vi "FaulhaberV3-Ascii_V1.vi"() -> (1 "searchnames":string[](array[string]), 2 "ID":u32[](array[numeric]), 3 "Faulhaber Objects":T3(array[cluster]))   [LabVIEW 2011] (continued)
  in  "?":string="<?xml version=\"1.0\" encoding=\"utf-8\"?>\n<ISO15745ProfileContainer xmlns=\"http://www.canopen.org/xml/1.0\" xmlns:xsi=\"http://www.w3.org/2001/XMLSchema-instance\" xsi:schemaLocation=\"http://www.canopen.org/xml/1.0 CANopen.xsd\">\n\t<ISO15745Profile>\n\t\t<ProfileHeader>\n\t\t\t<ProfileIdentification>CAN device profile</ProfileIdentification>\n\t\t\t<ProfileRevision>1</ProfileRevision>\n\t\t\t<ProfileName></ProfileName>\n\t\t\t<ProfileSource></ProfileSource>\n\t\t\t<ProfileClassID>Device</ProfileClassID>\n\t\t\t<ISO15745Reference>\n\t\t\t\t<ISO15745Part>1</ISO15745Part>\n\t\t\t\t<ISO15745Edition>1</ISO15745Edition>\n\t\t\t\t<ProfileTechnology>CANopen</ProfileTechnology>\n\t\t\t</ISO15745Reference>\n\t\t</ProfileHeader>\n\t\t<ProfileBody xsi:type=\"ProfileBody_Device_CANopen\" fileName=\"605.0161.01-O.xdd\" fileCreator=\"Dr. Fritz Faulhaber GmbH &amp; Co KG\" fileCreationDate=\"2024-11-08\" fileCreationTime=\"07:04:39\" fileModificationDate=\"2024-11-08\" fileModificationTime=\"07:04:39\" fileModifiedBy=\"Dr. Fritz Faulhaber GmbH &amp; Co KG\" fileVersion=\"1\" supportedLanguages=\"en\">\n\t\t\t<DeviceIdentity>\n\t\t\t\t<vendorName readOnly=\"true\">Dr. Fritz Faulhaber GmbH &amp; Co KG</vendorName>\n\t\t\t\t<vendorID readOnly=\"true\">327</vendorID>\n\t\t\t\t<vendorText readOnly=\"true\">\n\t\t\t\t\t<label lang=\"en\" />\n\t\t\t\t</vendorText>\n\t\t\t\t<deviceFamily readOnly=\"true\">\n\t\t\t\t\t<label lang=\"en\" />\n\t\t\t\t</deviceFamily>\n\t\t\t\t<productFamily readOnly=\"true\">MC V3.x</productFamily>\n\t\t\t\t<productName readOnly=\"true\">IMC *</productName>\n\t\t\t\t<productID readOnly=\"true\">016101</productID>\n\t\t\t\t<productText readOnly=\"true\">\n\t\t\t\t\t<description lang=\"en\">FileDescription=Faulhaber MC V3.x device description|EdsVersion=4.0|FileRevison=1|RevisionNum=0x00010000|</description>\n\t\t\t\t</productText>\n\t\t\t\t<orderNumber readOnly=\"true\">0</orderNumber>\n\t\t\t\t<version versionType=\"SW\" readOnly=\"true\"></version>\n\t\t\t\t<version versionType=\"FW\" readOnly=\"true\"></version>\n\t\t\t\t<version versionType=\"HW\" readOnly=\"true\"></version>\n\t\t\t\t<specificationRevision readOnly=\"true\"></specificationRevision>\n\t\t\t\t<instanceName readOnly=\"true\"></instanceName>\n\t\t\t</DeviceIdentity>\n\t\t\t<DeviceManager>\n\t\t\t\t<indicatorList>\n\t\t\t\t\t<LEDList>\n\t\t\t\t\t\t<LED LEDcolors=\"monocolor\" LEDtype=\"device\">\n\t\t\t\t\t\t\t<label lang=\"en\" />\n\t\t\t\t\t\t\t<LEDstate uniqueID=\"LED_State_1\" state=\"off\" LEDcolor=\"green\">\n\t\t\t\t\t\t\t\t<label lang=\"en\" />\n\t\t\t\t\t\t\t</LEDstate>\n\t\t\t\t\t\t</LED>\n\t\t\t\t\t</LEDList>\n\t\t\t\t</indicatorList>\n\t\t\t</DeviceManager>\n\t\t\t<DeviceFunction>\n\t\t\t\t<capabilities>\n\t\t\t\t\t<characteristicsList>\n\t\t\t\t\t\t<characteristic>\n\t\t\t\t\t\t\t<characteristicName>\n\t\t\t\t\t\t\t\t<label lang=\"en\" />\n\t\t\t\t\t\t\t</characteristicName>\n\t\t\t\t\t\t\t<characteristicContent>\n\t\t\t\t\t\t\t\t<label lang=\"en\" />\n\t\t\t\t\t\t\t</characteristicContent>\n\t\t\t\t\t\t</characteristic>\n\t\t\t\t\t</characteristicsList>\n\t\t\t\t</capabilities>\n\t\t\t</DeviceFunction>\n\t\t\t<ApplicationProcess>\n\t\t\t\t<parameterList>\n\t\t\t\t\t<parameter uniqueID=\"UID_PARAM_102901\" access=\"readWrite\">\n\t\t\t\t\t\t<label lang=\"en\">Communication error</label>\n\t\t\t\t\t\t<USINT />\n\t\t\t\t\t\t<denotation>\n\t\t\t\t\t\t\t<label lang=\"en\" />\n\t\t\t\t\t\t</denotation>\n\t\t\t\t\t\t<defaultValue value=\"0\" />\n\t\t\t\t\t\t<allowedValues>\n\t\t\t\t\t\t\t<range>\n\t\t\t\t\t\t\t\t<minValue value=\"0\" />\n\t\t\t\t\t\t\t\t<maxValue value=\"255\" />\n\t\t\t\t\t\t\t</range>\n\t\t\t\t\t\t\t<value value=\"0\" />\n\t\t\t\t\t\t\t<value value=\"1\" />\n\t\t\t\t\t\t\t<value value=\"2\" />\n\t\t\t\t\t\t</allowedValues>\n\t\t\t\t\t</parameter>\n\t\t\t\t\t<parameter uniqueID=\"UID_PARAM_230004\" access=\"readWrite\">\n\t\t\t\t\t\t<label lang=\"en\">Number of emulated digital inputs</label>\n\t\t\t\t\t\t<USINT />\n\t\t\t\t\t\t<denotation>\n\t\t\t\t\t\t\t<label lang=\"en\" />\n\t\t\t\t\t\t</denotation>\n\t\t\t\t\t\t<defaultValue value=\"0\" />\n\t\t\t\t\t\t<allowedValues>\n\t\t\t\t\t\t\t<range>\n\t\t\t\t\t\t\t\t<minValue value=\"0\" />\n\t\t\t\t\t\t\t\t<maxValue value=\"2\" />\n\t\t\t\t\t\t\t</range>\n\t\t\t\t\t\t\t<value value=\"0\" />\n\t\t\t\t\t\t\t<value value=\"1\" />\n\t\t\t\t\t\t\t<value value=\"2\" />\n\t\t\t\t\t\t</allowedValues>\n\t\t\t\t\t</parameter>\n\t\t\t\t\t<parameter uniqueID=\"UID_PARAM_231001\" access=\"readWrite\">\n\t\t\t\t\t\t<label lang=\"en\">Select lower limit switch inputs</label>\n\t\t\t\t\t\t<USINT />\n\t\t\t\t\t\t<denotation>\n\t\t\t\t\t\t\t<label lang=\"en\" />\n\t\t\t\t\t\t</denotation>\n\t\t\t\t\t\t<defaultValue value=\"0x0\" />\n\t\t\t\t\t\t<allowedValues>\n\t\t\t\t\t\t\t<range>\n\t\t\t\t\t\t\t\t<minValue value=\"0\" />\n\t\t\t\t\t\t\t\t<maxValue value=\"255\" />\n\t\t\t\t\t\t\t</range>\n\t\t\t\t\t\t\t<value value=\"0\" />\n\t\t\t\t\t\t\t<value value=\"1\" />\n\t\t\t\t\t\t\t<value value=\"2\" />\n\t\t\t\t\t\t\t<value value=\"4\" />\n\t\t\t\t\t\t\t<value value=\"8\" />\n\t\t\t\t\t\t\t<value value=\"16\" />\n\t\t\t\t\t\t\t<value value=\"32\" />\n\t\t\t\t\t\t\t<value value=\"64\" />\n\t\t\t\t\t\t\t<value value=\"128\" />\n\t\t\t\t\t\t</allowedValues>\n\t\t\t\t\t</parameter>\n\t\t\t\t\t<parameter uniqueID=\"UID_PARAM_231002\" access=\"readWrite\">\n\t\t\t\t\t\t<label lang=\"en\">Select upper limit switch inputs</label>\n\t\t\t\t\t\t<USINT />\n\t\t\t\t\t\t<denotation>\n\t\t\t\t\t\t\t<label lang=\"en\" />\n\t\t\t\t\t\t</denotation>\n\t\t\t\t\t\t<defaultValue value=\"0x0\" />\n\t\t\t\t\t\t<allowedValues>\n\t\t\t\t\t\t\t<range>\n\t\t\t\t\t\t\t\t<minValue value=\"0\" />\n\t\t\t\t\t\t\t\t<maxValue value=\"255\" />\n\t\t\t\t\t\t\t</range>\n\t\t\t\t\t\t\t<value value=\"0\" />\n\t\t\t\t\t\t\t<value value=\"1\" />\n\t\t\t\t\t\t\t<value value=\"2\" />\n\t\t\t\t\t\t\t<value value=\"4\" />\n\t\t\t\t\t\t\t<value value=\"8\" />\n\t\t\t\t\t\t\t<value value=\"16\" />\n\t\t\t\t\t\t\t<value value=\"32\" />\n\t\t\t\t\t\t\t<value value=\"64\" />\n\t\t\t\t\t\t\t<value value=\"128\" />\n\t\t\t\t\t\t</allowedValues>\n\t\t\t\t\t</parameter>\n\t\t\t\t\t<parameter uniqueID=\"UID_PARAM_231003\" access=\"readWrite\">\n\t\t\t\t\t\t<label lang=\"en\">Limit switch option code</label>\n\t\t\t\t\t\t<INT />\n\t\t\t\t\t\t<denotation>\n\t\t\t\t\t\t\t<label lang=\"en\" />\n\t\t\t\t\t\t</denotation>\n\t\t\t\t\t\t<defaultValue value=\"1\" />\n\t\t\t\t\t\t<allowedValues>\n\t\t\t\t\t\t\t<range>\n\t\t\t\t\t\t\t\t<minValue value=\"-32768\" />\n\t\t\t\t\t\t\t\t<maxValue value=\"32767\" />\n\t\t\t\t\t\t\t</range>\n\t\t\t\t\t\t\t<value value=\"0\" />\n\t\t\t\t\t\t\t<value value=\"1\" />\n\t\t\t\t\t\t\t<value value=\"2\" />\n\t\t\t\t\t\t\t<value value=\"3\" />\n\t\t\t\t\t\t\t<value value=\"4\" />\n\t\t\t\t\t\t</allowedValues>\n\t\t\t\t\t</parameter>\n\t\t\t\t\t<parameter uniqueID=\"UID_PARAM_231006\" access=\"readWrite\">\n\t\t\t\t\t\t<label lang=\"en\">Select stop input</label>\n\t\t\t\t\t\t<USINT />\n\t\t\t\t\t\t<denotation>\n\t\t\t\t\t\t\t<label lang=\"en\" />\n\t\t\t\t\t\t</denotation>\n\t\t\t\t\t\t<defaultValue value=\"0x0\" />\n\t\t\t\t\t\t<allowedValues>\n\t\t\t\t\t\t\t<range>\n\t\t\t\t\t\t\t\t<minValue value=\"0\" />\n\t\t\t\t\t\t\t\t<maxValue value=\"255\" />\n\t\t\t\t\t\t\t</range>\n\t\t\t\t\t\t\t<value value=\"0\" />\n\t\t\t\t\t\t\t<value value=\"1\" />\n\t\t\t\t\t\t\t<value value=\"2\" />\n\t\t\t\t\t\t\t<value value=\"4\" />\n\t\t\t\t\t\t\t<value value=\"8\" />\n\t\t\t\t\t\t\t<value value=\"16\" />\n\t\t\t\t\t\t\t<value value=\"32\" />\n\t\t\t\t\t\t\t<value value=\"64\" />\n\t\t\t\t\t\t\t<value value=\"128\" />\n\t\t\t\t\t\t</allowedValues>\n\t\t\t\t\t</parameter>\n\t\t\t\t\t<parameter uniqueID=\"UID_PARAM_231011\" access=\"readWrite\">\n\t\t\t\t\t\t<label lang=\"en\">Input threshold level</label>\n\t\t\t\t\t\t<USINT />\n\t\t\t\t\t\t<denotation>\n\t\t\t\t\t\t\t<label lang=\"en\" />\n\t\t\t\t\t\t</denotation>\n\t\t\t\t\t\t<defaultValue value=\"0\" />\n\t\t\t\t\t\t<allowedValues>\n\t\t\t\t\t\t\t<range>\n\t\t\t\t\t\t\t\t<minValue value=\"0\" />\n\t\t\t\t\t\t\t\t<maxValue value=\"1\" />\n\t\t\t\t\t\t\t</range>\n\t\t\t\t\t\t\t<value value=\"0\" />\n\t\t\t\t\t\t\t<value value=\"1\" />\n\t\t\t\t\t\t</allowedValues>\n\t\t\t\t\t</parameter>\n\t\t\t\t\t<parameter uniqueID=\"UID_PARAM_23130A\" access=\"readWriteInput\">\n\t\t\t\t\t\t<label lang=\"en\">AnIn 1 enable virtual input</label>\n\t\t\t\t\t\t<USINT />\n\t\t\t\t\t\t<denotation>\n\t\t\t\t\t\t\t<label lang=\"en\" />\n\t\t\t\t\t\t</denotation>\n\t\t\t\t\t\t<defaultValue value=\"0\" />\n\t\t\t\t\t\t<allowedValues>\n\t\t\t\t\t\t\t<range>\n\t\t\t\t\t\t\t\t<minValue value=\"0\" />\n\t\t\t\t\t\t\t\t<maxValue value=\"255\" />\n\t\t\t\t\t\t\t</range>\n\t\t\t\t\t\t\t<value value=\"0\" />\n\t\t\t\t\t\t\t<value value=\"1\" />\n\t\t\t\t\t\t</allowedValues>\n\t\t\t\t\t</parameter>\n\t\t\t\t\t<parameter uniqueID=\"UID_PARAM_23131A\" access=\"readWriteInput\">\n\t\t\t\t\t\t<label lang=\"en\">AnIn 2 enable virtual input</label>\n\t\t\t\t\t\t<USINT />\n\t\t\t\t\t\t<denotation>\n\t\t\t\t\t\t\t<label lang=\"en\" />\n\t\t\t\t\t\t</denotation>\n\t\t\t\t\t\t<defaultValue value=\"0\" />\n\t\t\t\t\t\t<allowedValues>\n\t\t\t\t\t\t\t<range>\n\t\t\t\t\t\t\t\t<minValue value=\"0\" />\n\t\t\t\t\t\t\t\t<maxValue value=\"255\" />\n\t\t\t\t\t\t\t</range>\n\t\t\t\t\t\t\t<value value=\"0\" />\n\t\t\t\t\t\t\t<value value=\"1\" />\n\t\t\t\t\t\t</allowedValues>\n\t\t\t\t\t</parameter>\n\t\t\t\t\t<parameter uniqueID=\"UID_PARAM_231701\" access=\"readWrite\">\n\t\t\t\t\t\t<label lang=\"en\">Digital input pin</label>\n\t\t\t\t\t\t<USINT />\n\t\t\t\t\t\t<denotation>\n\t\t\t\t\t\t\t<label lang=\"en\" />\n\t\t\t\t\t\t</denotation>\n\t\t\t\t\t\t<defaultValue value=\"0\" />\n\t\t\t\t\t\t<allowedValues>\n\t\t\t\t\t\t\t<range>\n\t\t\t\t\t\t\t\t<minValue value=\"0\" />\n\t\t\t\t\t\t\t\t<maxValue value=\"2\" />\n\t\t\t\t\t\t\t</range>\n\t\t\t\t\t\t\t<value value=\"0\" />\n\t\t\t\t\t\t\t<value value=\"1\" />\n\t\t\t\t\t\t\t<value value=\"2\" />\n\t\t\t\t\t\t</allowedValues>\n\t\t\t\t\t</parameter>\n\t\t\t\t\t<parameter uniqueID=\"UID_PARAM_232801\" access=\"read\">\n\t\t\t\t\t\t<label lang=\"en\">Controller type</label>\n\t\t\t\t\t\t<USINT />\n\t\t\t\t\t\t<denotation>\n\t\t\t\t\t\t\t<label lang=\"en\" />\n\t\t\t\t\t\t</denotation>\n\t\t\t\t\t\t<allowedValues>\n\t\t\t\t\t\t\t<value value=\"0\" />\n\t\t\t\t\t\t\t<value value=\"1\" />\n\t\t\t\t\t\t</allowedValues>\n\t\t\t\t\t</parameter>\n\t\t\t\t\t<parameter uniqueID=\"UID_PARAM_23290B\" access=\"read\">\n\t\t\t\t\t\t<label lang=\"en\">Motor type</label>\n\t\t\t\t\t\t<USINT />\n\t\t\t\t\t\t<denotation>\n\t\t\t\t\t\t\t<label lang=\"en\" />\n\t\t\t\t\t\t</denotation>\n\t\t\t\t\t\t<allowedValues>\n\t\t\t\t\t\t\t<value value=\"0\" />\n\t\t\t\t\t\t\t<value value=\"1\" />\n\t\t\t\t\t\t</allowedValues>\n\t\t\t\t\t</parameter>\n\t\t\t\t\t<parameter uniqueID=\"UID_PARAM_233001\" access=\"readWriteInput\">\n\t\t\t\t\t\t<label lang=\"en\">Actual commutation angle source</label>\n\t\t\t\t\t\t<USINT />\n\t\t\t\t\t\t<denotation>\n\t\t\t\t\t\t\t<label lang=\"en\" />\n\t\t\t\t\t\t</denotation>\n\t\t\t\t\t\t<defaultValue value=\"0\" />\n\t\t\t\t\t\t<allowedValues>\n\t\t\t\t\t\t\t<range>\n\t\t\t\t\t\t\t\t<minValue value=\"0\" />\n\t\t\t\t\t\t\t\t<maxValue value=\"15\" />\n\t\t\t\t\t\t\t</range>\n\t\t\t\t\t\t\t<value value=\"0\" />\n\t\t\t\t\t\t\t<value value=\"1\" />\n\t\t\t\t\t\t\t<value value=\"2\" />\n\t\t\t\t\t\t\t<value value=\"3\" />\n\t\t\t\t\t\t\t<value value=\"4\" />\n\t\t\t\t\t\t\t<value value=\"5\" />\n\t\t\t\t\t\t\t<value value=\"15\" />\n\t\t\t\t\t\t</allowedValues>\n\t\t\t\t\t</parameter>\n\t\t\t\t\t<parameter uniqueID=\"UID_PARAM_233002\" access=\"readWriteInput\">\n\t\t\t\t\t\t<label lang=\"en\">Actual velocity source</label>\n\t\t\t\t\t\t<USINT />\n\t\t\t\t\t\t<denotation>\n\t\t\t\t\t\t\t<label lang=\"en\" />\n\t\t\t\t\t\t</denotation>\n\t\t\t\t\t\t<defaultValue value=\"0\" />\n\t\t\t\t\t\t<allowedValues>\n\t\t\t\t\t\t\t<range>\n\t\t\t\t\t\t\t\t<minValue value=\"0\" />\n\t\t\t\t\t\t\t\t<maxValue value=\"24\" />\n\t\t\t\t\t\t\t</range>\n\t\t\t\t\t\t\t<value value=\"0\" />\n\t\t\t\t\t\t\t<value value=\"1\" />\n\t\t\t\t\t\t\t<value value=\"2\" />\n\t\t\t\t\t\t\t<value value=\"3\" />\n\t\t\t\t\t\t\t<value value=\"4\" />\n\t\t\t\t\t\t\t<value value=\"5\" />\n\t\t\t\t\t\t\t<value value=\"6\" />\n\t\t\t\t\t\t\t<value value=\"7\" />\n\t\t\t\t\t\t\t<value value=\"8\" />\n\t\t\t\t\t\t\t<value value=\"13\" />\n\t\t\t\t\t\t\t<value value=\"23\" />\n\t\t\t\t\t\t\t<value value=\"24\" />\n\t\t\t\t\t\t</allowedValues>\n\t\t\t\t\t</parameter>\n\t\t\t\t\t<parameter uniqueID=\"UID_PARAM_233003\" access=\"readWriteInput\">\n\t\t\t\t\t\t<label lang=\"en\">Actual position source</label>\n\t\t\t\t\t\t<USINT />\n\t\t\t\t\t\t<denotation>\n\t\t\t\t\t\t\t<label lang=\"en\" />\n\t\t\t\t\t\t</denotation>\n\t\t\t\t\t\t<defaultValue value=\"0\" />\n\t\t\t\t\t\t<allowedValues>\n\t\t\t\t\t\t\t<range>\n\t\t\t\t\t\t\t\t<minValue value=\"0\" />\n\t\t\t\t\t\t\t\t<maxValue value=\"13\" />\n\t\t\t\t\t\t\t</range>\n\t\t\t\t\t\t\t<value value=\"0\" />\n\t\t\t\t\t\t\t<value value=\"1\" />\n\t\t\t\t\t\t\t<value value=\"2\" />\n\t\t\t\t\t\t\t<value value=\"3\" />\n\t\t\t\t\t\t\t<value value=\"4\" />\n\t\t\t\t\t\t\t<value value=\"5\" />\n\t\t\t\t\t\t\t<value value=\"6\" />\n\t\t\t\t\t\t\t<value value=\"7\" />\n\t\t\t\t\t\t\t<value value=\"8\" />\n\t\t\t\t\t\t\t<value value=\"13\" />\n\t\t\t\t\t\t</allowedValues>\n\t\t\t\t\t</parameter>\n\t\t\t\t\t<parameter uniqueID=\"UID_PARAM_233101\" access=\"readWriteInput\">\n\t\t\t\t\t\t<label lang=\"en\">Target voltage source</label>\n\t\t\t\t\t\t<USINT />\n\t\t\t\t\t\t<denotation>\n\t\t\t\t\t\t\t<label lang=\"en\" />\n\t\t\t\t\t\t</denotation>\n\t\t\t\t\t\t<defaultValue value=\"0\" />\n\t\t\t\t\t\t<allowedValues>\n\t\t\t\t\t\t\t<range>\n\t\t\t\t\t\t\t\t<minValue value=\"0\" />\n\t\t\t\t\t\t\t\t<maxValue value=\"10\" />\n\t\t\t\t\t\t\t</range>\n\t\t\t\t\t\t\t<value value=\"0\" />\n\t\t\t\t\t\t\t<value value=\"1\" />\n\t\t\t\t\t\t\t<value value=\"2\" />\n\t\t\t\t\t\t\t<value value=\"7\" />\n\t\t\t\t\t\t</allowedValues>\n\t\t\t\t\t</parameter>\n\t\t\t\t\t<parameter uniqueID=\"UID_PARAM_233102\" access=\"readWriteInput\">\n\t\t\t\t\t\t<label lang=\"en\">Target current source</label>\n\t\t\t\t\t\t<USINT />\n\t\t\t\t\t\t<denotation>\n\t\t\t\t\t\t\t<label lang=\"en\" />\n\t\t\t\t\t\t</denotation>\n\t\t\t\t\t\t<defaultValue value=\"0\" />\n\t\t\t\t\t\t<allowedValues>\n\t\t\t\t\t\t\t<range>\n\t\t\t\t\t\t\t\t<minValue value=\"0\" />\n\t\t\t\t\t\t\t\t<maxValue value=\"10\" />\n\t\t\t\t\t\t\t</range>\n\t\t\t\t\t\t\t<value value=\"0\" />\n\t\t\t\t\t\t\t<value value=\"1\" />\n\t\t\t\t\t\t\t<value value=\"2\" />\n\t\t\t\t\t\t\t<value value=\"7\" />\n\t\t\t\t\t\t</allowedValues>\n\t\t\t\t\t</parameter>\n\t\t\t\t\t<parameter uniqueID=\"UID_PARAM_233103\" access=\"readWriteInput\">\n\t\t\t\t\t\t<label lang=\"en\">Target velocity source</label>\n\t\t\t\t\t\t<USINT />\n\t\t\t\t\t\t<denotation>\n\t\t\t\t\t\t\t<label lang=\"en\" />\n\t\t\t\t\t\t</denotation>\n\t\t\t\t\t\t<defaultValue value=\"0\" />\n\t\t\t\t\t\t<allowedValues>\n\t\t\t\t\t\t\t<range>\n\t\t\t\t\t\t\t\t<minValue value=\"0\" />\n\t\t\t\t\t\t\t\t<maxValue value=\"10\" />\n\t\t\t\t\t\t\t</range>\n\t\t\t\t\t\t\t<value value=\"0\" />\n\t\t\t\t\t\t\t<value value=\"1\" />\n\t\t\t\t\t\t\t<value value=\"2\" />\n\t\t\t\t\t\t\t<value value=\"7\" />\n\t\t\t\t\t\t\t<value value=\"8\" />\n\t\t\t\t\t\t\t<value value=\"9\" />\n\t\t\t\t\t\t</allowedValues>\n\t\t\t\t\t</parameter>\n\t\t\t\t\t<parameter uniqueID=\"UID_PARAM_233104\" access=\"readWriteInput\">\n\t\t\t\t\t\t<label lang=\"en\">Target position source</label>\n\t\t\t\t\t\t<USINT />\n\t\t\t\t\t\t<denotation>\n\t\t\t\t\t\t\t<label lang=\"en\" />\n\t\t\t\t\t\t</denotation>\n\t\t\t\t\t\t<defaultValue value=\"0\" />\n\t\t\t\t\t\t<allowedValues>\n\t\t\t\t\t\t\t<range>\n\t\t\t\t\t\t\t\t<minValue value=\"0\" />\n\t\t\t\t\t\t\t\t<maxValue value=\"10\" />\n\t\t\t\t\t\t\t</range>\n\t\t\t\t\t\t\t<value value=\"0\" />\n\t\t\t\t\t\t\t<value value=\"1\" />\n\t\t\t\t\t\t\t<value value=\"2\" />\n\t\t\t\t\t\t\t<value value=\"7\" />\n\t\t\t\t\t\t\t<value value=\"8\" />\n\t\t\t\t\t\t\t<value value=\"9\" />\n\t\t\t\t\t\t</allowedValues>\n\t\t\t\t\t</parameter>\n\t\t\t\t\t<parameter uniqueID=\"UID_PARAM_234001\" access=\"readWrite\">\n\t\t\t\t\t\t<label lang=\"en\">Commutation type</label>\n\t\t\t\t\t\t<USINT />\n\t\t\t\t\t\t<denotation>\n\t\t\t\t\t\t\t<label lang=\"en\" />\n\t\t\t\t\t\t</denotation>\n\t\t\t\t\t\t<defaultValue value=\"3\" />\n\t\t\t\t\t\t<allowedValues>\n\t\t\t\t\t\t\t<range>\n\t\t\t\t\t\t\t\t<minValue value=\"0\" />\n\t\t\t\t\t\t\t\t<maxValue value=\"255\" />\n\t\t\t\t\t\t\t</range>\n\t\t\t\t\t\t\t<value value=\"1\" />\n\t\t\t\t\t\t\t<value value=\"2\" />\n\t\t\t\t\t\t\t<value value=\"3\" />\n\t\t\t\t\t\t\t<value value=\"4\" />\n\t\t\t\t\t\t\t<value value=\"5\" />\n\t\t\t\t\t\t\t<value value=\"15\" />\n\t\t\t\t\t\t</allowedValues>\n\t\t\t\t\t</parameter>\n\t\t\t\t\t<parameter uniqueID=\"UID_PARAM_234406\" access=\"readWriteInput\">\n\t\t\t\t\t\t<label lang=\"en\">Integral part option</label>\n\t\t\t\t\t\t<USINT />\n\t\t\t\t\t\t<denotation>\n\t\t\t\t\t\t\t<label lang=\"en\" />\n\t\t\t\t\t\t</denotation>\n\t\t\t\t\t\t<defaultValue value=\"0\" />\n\t\t\t\t\t\t<allowedValues>\n\t\t\t\t\t\t\t<range>\n\t\t\t\t\t\t\t\t<minValue value=\"0\" />\n\t\t\t\t\t\t\t\t<maxValue value=\"2\" />\n\t\t\t\t\t\t\t</range>\n\t\t\t\t\t\t\t<value value=\"0\" />\n\t\t\t\t\t\t\t<value value=\"1\" />\n\t\t\t\t\t\t\t<value value=\"2\" />\n\t\t\t\t\t\t</allowedValues>\n\t\t\t\t\t</parameter>\n\t\t\t\t\t<parameter uniqueID=\"UID_PARAM_234602\" access=\"readWriteInput\">\n\t\t\t\t\t\t<label lang=\"en\">Setpoint filter enable</label>\n\t\t\t\t\t\t<USINT />\n\t\t\t\t\t\t<denotation>\n\t\t\t\t\t\t\t<label lang=\"en\" />\n\t\t\t\t\t\t</denotation>\n\t\t\t\t\t\t<allowedValues>\n\t\t\t\t\t\t\t<range>\n\t\t\t\t\t\t\t\t<minValue value=\"0\" />\n\t\t\t\t\t\t\t\t<maxValue value=\"255\" />\n\t\t\t\t\t\t\t</range>\n\t\t\t\t\t\t\t<value value=\"0\" />\n\t\t\t\t\t\t\t<value value=\"1\" />\n\t\t\t\t\t\t</allowedValues>\n\t\t\t\t\t</parameter>\n\t\t\t\t\t<parameter uniqueID=\"UID_PARAM_237301\" access=\"readWrite\">\n\t\t\t\t\t\t<label lang=\"en\">Event trigger event selection</label>\n\t\t\t\t\t\t<UINT />\n\t\t\t\t\t\t<denotation>\n\t\t\t\t\t\t\t<label lang=\"en\" />\n\t\t\t\t\t\t</denotation>\n\t\t\t\t\t\t<defaultValue value=\"0\" />\n\t\t\t\t\t\t<allowedValues>\n\t\t\t\t\t\t\t<range>\n\t\t\t\t\t\t\t\t<minValue value=\"0\" />\n\t\t\t\t\t\t\t\t<maxValue value=\"65535\" />\n\t\t\t\t\t\t\t</range>\n\t\t\t\t\t\t\t<value value=\"0\" />\n\t\t\t\t\t\t\t<value value=\"1\" />\n\t\t\t\t\t\t\t<value value=\"2\" />\n\t\t\t\t\t\t\t<value value=\"3\" />\n\t\t\t\t\t\t</allowedValues>\n\t\t\t\t\t</parameter>\n\t\t\t\t\t<parameter uniqueID=\"UID_PARAM_237805\" access=\"readWriteInput\">\n\t\t\t\t\t\t<label lang=\"en\">Channel 1 start event selection</label>\n\t\t\t\t\t\t<USINT />\n\t\t\t\t\t\t<denotation>\n\t\t\t\t\t\t\t<label lang=\"en\" />\n\t\t\t\t\t\t</denotation>\n\t\t\t\t\t\t<defaultValue value=\"0\" />\n\t\t\t\t\t\t<allowedValues>\n\t\t\t\t\t\t\t<range>\n\t\t\t\t\t\t\t\t<minValue value=\"0\" />\n\t\t\t\t\t\t\t\t<maxValue value=\"255\" />\n\t\t\t\t\t\t\t</range>\n\t\t\t\t\t\t\t<value value=\"0\" />\n\t\t\t\t\t\t\t<value value=\"1\" />\n\t\t\t\t\t\t\t<value value=\"2\" />\n\t\t\t\t\t\t\t<value value=\"3\" />\n\t\t\t\t\t\t\t<value value=\"4\" />\n\t\t\t\t\t\t\t<value value=\"5\" />\n\t\t\t\t\t\t\t<value value=\"6\" />\n\t\t\t\t\t\t\t<value value=\"7\" />\n\t\t\t\t\t\t\t<value value=\"8\" />\n\t\t\t\t\t\t\t<value value=\"9\" />\n\t\t\t\t\t\t\t<value value=\"10\" />\n\t\t\t\t\t\t\t<value value=\"11\" />\n\t\t\t\t\t\t\t<value value=\"13\" />\n\t\t\t\t\t\t\t<value value=\"14\" />\n\t\t\t\t\t\t\t<value value=\"15\" />\n\t\t\t\t\t\t</allowedValues>\n\t\t\t\t\t</parameter>\n\t\t\t\t\t<parameter uniqueID=\"UID_PARAM_237806\" access=\"readWriteInput\">\n\t\t\t\t\t\t<label lang=\"en\">Channel 1 update event selection</label>\n\t\t\t\t\t\t<USINT />\n\t\t\t\t\t\t<denotation>\n\t\t\t\t\t\t\t<label lang=\"en\" />\n\t\t\t\t\t\t</denotation>\n\t\t\t\t\t\t<defaultValue value=\"0\" />\n\t\t\t\t\t\t<allowedValues>\n\t\t\t\t\t\t\t<range>\n\t\t\t\t\t\t\t\t<minValue value=\"0\" />\n\t\t\t\t\t\t\t\t<maxValue value=\"255\" />\n\t\t\t\t\t\t\t</range>\n\t\t\t\t\t\t\t<value value=\"0\" />\n\t\t\t\t\t\t\t<value value=\"1\" />\n\t\t\t\t\t\t\t<value value=\"2\" />\n\t\t\t\t\t\t\t<value value=\"3\" />\n\t\t\t\t\t\t\t<value value=\"4\" />\n\t\t\t\t\t\t\t<value value=\"5\" />\n\t\t\t\t\t\t\t<value value=\"6\" />\n\t\t\t\t\t\t\t<value value=\"7\" />\n\t\t\t\t\t\t\t<value value=\"8\" />\n\t\t\t\t\t\t\t<value value=\"9\" />\n\t\t\t\t\t\t\t<value value=\"10\" />\n\t\t\t\t\t\t\t<value value=\"11\" />\n\t\t\t\t\t\t\t<value value=\"13\" />\n\t\t\t\t\t\t\t<value value=\"14\" />\n\t\t\t\t\t\t\t<value value=\"15\" />\n\t\t\t\t\t\t</allowedValues>\n\t\t\t\t\t</parameter>\n\t\t\t\t\t<parameter uniqueID=\"UID_PARAM_237905\" access=\"readWriteInput\">\n\t\t\t\t\t\t<label lang=\"en\">Channel 2 startevent selection</label>\n\t\t\t\t\t\t<USINT />\n\t\t\t\t\t\t<denotation>\n\t\t\t\t\t\t\t<label lang=\"en\" />\n\t\t\t\t\t\t</denotation>\n\t\t\t\t\t\t<defaultValue value=\"0\" />\n\t\t\t\t\t\t<allowedValues>\n\t\t\t\t\t\t\t<range>\n\t\t\t\t\t\t\t\t<minValue value=\"0\" />\n\t\t\t\t\t\t\t\t<maxValue value=\"255\" />\n\t\t\t\t\t\t\t</range>\n\t\t\t\t\t\t\t<value value=\"0\" />\n\t\t\t\t\t\t\t<value value=\"1\" />\n\t\t\t\t\t\t\t<value value=\"2\" />\n\t\t\t\t\t\t\t<value value=\"3\" />\n\t\t\t\t\t\t\t<value value=\"4\" />\n\t\t\t\t\t\t\t<value value=\"5\" />\n\t\t\t\t\t\t\t<value value=\"6\" />\n\t\t\t\t\t\t\t<value value=\"7\" />\n\t\t\t\t\t\t\t<value value=\"8\" />\n\t\t\t\t\t\t\t<value value=\"9\" />\n\t\t\t\t\t\t\t<value value=\"10\" />\n\t\t\t\t\t\t\t<value value=\"11\" />\n\t\t\t\t\t\t\t<value value=\"12\" />\n\t\t\t\t\t\t\t<value value=\"14\" />\n\t\t\t\t\t\t\t<value value=\"15\" />\n\t\t\t\t\t\t</allowedValues>\n\t\t\t\t\t</parameter>\n\t\t\t\t\t<parameter uniqueID=\"UID_PARAM_237906\" access=\"readWriteInput\">\n\t\t\t\t\t\t<label lang=\"en\">Channel 2 update event selection</label>\n\t\t\t\t\t\t<USINT />\n\t\t\t\t\t\t<denotation>\n\t\t\t\t\t\t\t<label lang=\"en\" />\n\t\t\t\t\t\t</denotation>\n\t\t\t\t\t\t<defaultValue value=\"0\" />\n\t\t\t\t\t\t<allowedValues>\n\t\t\t\t\t\t\t<range>\n\t\t\t\t\t\t\t\t<minValue value=\"0\" />\n\t\t\t\t\t\t\t\t<maxValue value=\"255\" />\n\t\t\t\t\t\t\t</range>\n\t\t\t\t\t\t\t<value value=\"0\" />\n\t\t\t\t\t\t\t<value value=\"1\" />\n\t\t\t\t\t\t\t<value value=\"2\" />\n\t\t\t\t\t\t\t<value value=\"3\" />\n\t\t\t\t\t\t\t<value value=\"4\" />\n\t\t\t\t\t\t\t<value value=\"5\" />\n\t\t\t\t\t\t\t<value value=\"6\" />\n\t\t\t\t\t\t\t<value value=\"7\" />\n\t\t\t\t\t\t\t<value value=\"8\" />\n\t\t\t\t\t\t\t<value value=\"9\" />\n\t\t\t\t\t\t\t<value value=\"10\" />\n\t\t\t\t\t\t\t<value value=\"11\" />\n\t\t\t\t\t\t\t<value value=\"12\" />\n\t\t\t\t\t\t\t<value value=\"14\" />\n\t\t\t\t\t\t\t<value value=\"15\" />\n\t\t\t\t\t\t</allowedValues>\n\t\t\t\t\t</parameter>\n\t\t\t\t\t<parameter uniqueID=\"UID_PARAM_237A05\" access=\"readWriteInput\">\n\t\t\t\t\t\t<label lang=\"en\">Channel 3 start event selection</label>\n\t\t\t\t\t\t<USINT />\n\t\t\t\t\t\t<denotation>\n\t\t\t\t\t\t\t<label lang=\"en\" />\n\t\t\t\t\t\t</denotation>\n\t\t\t\t\t\t<defaultValue value=\"0\" />\n\t\t\t\t\t\t<allowedValues>\n\t\t\t\t\t\t\t<range>\n\t\t\t\t\t\t\t\t<minValue value=\"0\" />\n\t\t\t\t\t\t\t\t<maxValue value=\"255\" />\n\t\t\t\t\t\t\t</range>\n\t\t\t\t\t\t\t<value value=\"0\" />\n\t\t\t\t\t\t\t<value value=\"1\" />\n\t\t\t\t\t\t\t<value value=\"2\" />\n\t\t\t\t\t\t\t<value value=\"3\" />\n\t\t\t\t\t\t\t<value value=\"4\" />\n\t\t\t\t\t\t\t<value value=\"5\" />\n\t\t\t\t\t\t\t<value value=\"6\" />\n\t\t\t\t\t\t\t<value value=\"7\" />\n\t\t\t\t\t\t\t<value value=\"8\" />\n\t\t\t\t\t\t\t<value value=\"9\" />\n\t\t\t\t\t\t\t<value value=\"10\" />\n\t\t\t\t\t\t\t<value value=\"11\" />\n\t\t\t\t\t\t\t<value value=\"12\" />\n\t\t\t\t\t\t\t<value value=\"13\" />\n\t\t\t\t\t\t\t<value value=\"15\" />\n\t\t\t\t\t\t</allowedValues>\n\t\t\t\t\t</parameter>\n\t\t\t\t\t<parameter uniqueID=\"UID_PARAM_237A06\" access=\"readWriteInput\">\n\t\t\t\t\t\t<label lang=\"en\">Channel 3 update event selection</label>\n\t\t\t\t\t\t<USINT />\n\t\t\t\t\t\t<denotation>\n\t\t\t\t\t\t\t<label lang=\"en\" />\n\t\t\t\t\t\t</denotation>\n\t\t\t\t\t\t<defaultValue value=\"0\" />\n\t\t\t\t\t\t<allowedValues>\n\t\t\t\t\t\t\t<range>\n\t\t\t\t\t\t\t\t<minValue value=\"0\" />\n\t\t\t\t\t\t\t\t<maxValue value=\"255\" />\n\t\t\t\t\t\t\t</range>\n\t\t\t\t\t\t\t<value value=\"0\" />\n\t\t\t\t\t\t\t<value value=\"1\" />\n\t\t\t\t\t\t\t<value value=\"2\" />\n\t\t\t\t\t\t\t<value value=\"3\" />\n\t\t\t\t\t\t\t<value value=\"4\" />\n\t\t\t\t\t\t\t<value value=\"5\" />\n\t\t\t\t\t\t\t<value value=\"6\" />\n\t\t\t\t\t\t\t<value value=\"7\" />\n\t\t\t\t\t\t\t<value value=\"8\" />\n\t\t\t\t\t\t\t<value value=\"9\" />\n\t\t\t\t\t\t\t<value value=\"10\" />\n\t\t\t\t\t\t\t<value value=\"11\" />\n\t\t\t\t\t\t\t<value value=\"12\" />\n\t\t\t\t\t\t\t<value value=\"13\" />\n\t\t\t\t\t\t\t<value value=\"15\" />\n\t\t\t\t\t\t</allowedValues>\n\t\t\t\t\t</parameter>\n\t\t\t\t\t<parameter uniqueID=\"UID_PARAM_237B05\" access=\"readWriteInput\">\n\t\t\t\t\t\t<label lang=\"en\">Channel 4 start event selection</label>\n\t\t\t\t\t\t<USINT />\n\t\t\t\t\t\t<denotation>\n\t\t\t\t\t\t\t<label lang=\"en\" />\n\t\t\t\t\t\t</denotation>\n\t\t\t\t\t\t<defaultValue value=\"0\" />\n\t\t\t\t\t\t<allowedValues>\n\t\t\t\t\t\t\t<range>\n\t\t\t\t\t\t\t\t<minValue value=\"0\" />\n\t\t\t\t\t\t\t\t<maxValue value=\"255\" />\n\t\t\t\t\t\t\t</range>\n\t\t\t\t\t\t\t<value value=\"0\" />\n\t\t\t\t\t\t\t<value value=\"1\" />\n\t\t\t\t\t\t\t<value value=\"2\" />\n\t\t\t\t\t\t\t<value value=\"3\" />\n\t\t\t\t\t\t\t<value value=\"4\" />\n\t\t\t\t\t\t\t<value value=\"5\" />\n\t\t\t\t\t\t\t<value value=\"6\" />\n\t\t\t\t\t\t\t<value value=\"7\" />\n\t\t\t\t\t\t\t<value value=\"8\" />\n\t\t\t\t\t\t\t<value value=\"9\" />\n\t\t\t\t\t\t\t<value value=\"10\" />\n\t\t\t\t\t\t\t<value value=\"11\" />\n\t\t\t\t\t\t\t<value value=\"12\" />\n\t\t\t\t\t\t\t<value value=\"13\" />\n\t\t\t\t\t\t\t<value value=\"14\" />\n\t\t\t\t\t\t</allowedValues>\n\t\t\t\t\t</parameter>\n\t\t\t\t\t<parameter uniqueID=\"UID_PARAM_237B06\" access=\"readWriteInput\">\n\t\t\t\t\t\t<label lang=\"en\">Channel 4 update event selection</label>\n\t\t\t\t\t\t<USINT />\n\t\t\t\t\t\t<denotation>\n\t\t\t\t\t\t\t<label lang=\"en\" />\n\t\t\t\t\t\t</denotation>\n\t\t\t\t\t\t<defaultValue value=\"0\" />\n\t\t\t\t\t\t<allowedValues>\n\t\t\t\t\t\t\t<range>\n\t\t\t\t\t\t\t\t<minValue value=\"0\" />\n\t\t\t\t\t\t\t\t<maxValue value=\"255\" />\n\t\t\t\t\t\t\t</range>\n\t\t\t\t\t\t\t<value value=\"0\" />\n\t\t\t\t\t\t\t<value value=\"1\" />\n\t\t\t\t\t\t\t<value value=\"2\" />\n\t\t\t\t\t\t\t<value value=\"3\" />\n\t\t\t\t\t\t\t<value value=\"4\" />\n\t\t\t\t\t\t\t<value value=\"5\" />\n\t\t\t\t\t\t\t<value value=\"6\" />\n\t\t\t\t\t\t\t<value value=\"7\" />\n\t\t\t\t\t\t\t<value value=\"8\" />\n\t\t\t\t\t\t\t<value value=\"9\" />\n\t\t\t\t\t\t\t<value value=\"10\" />\n\t\t\t\t\t\t\t<value value=\"11\" />\n\t\t\t\t\t\t\t<value value=\"12\" />\n\t\t\t\t\t\t\t<value value=\"13\" />\n\t\t\t\t\t\t\t<value value=\"14\" />\n\t\t\t\t\t\t</allowedValues>\n\t\t\t\t\t</parameter>\n\t\t\t\t\t<parameter uniqueID=\"UID_PARAM_240001\" access=\"readWrite\">\n\t\t\t\t\t\t<label lang=\"en\">CAN rate</label>\n\t\t\t\t\t\t<USINT />\n\t\t\t\t\t\t<denotation>\n\t\t\t\t\t\t\t<label lang=\"en\" />\n\t\t\t\t\t\t</denotation>\n\t\t\t\t\t\t<defaultValue value=\"9\" />\n\t\t\t\t\t\t<allowedValues>\n\t\t\t\t\t\t\t<range>\n\t\t\t\t\t\t\t\t<minValue value=\"0\" />\n\t\t\t\t\t\t\t\t<maxValue value=\"9\" />\n\t\t\t\t\t\t\t</range>\n\t\t\t\t\t\t\t<value value=\"0\" />\n\t\t\t\t\t\t\t<value value=\"2\" />\n\t\t\t\t\t\t\t<value value=\"3\" />\n\t\t\t\t\t\t\t<value value=\"4\" />\n\t\t\t\t\t\t\t<value value=\"5\" />\n\t\t\t\t\t\t\t<value value=\"6\" />\n\t\t\t\t\t\t\t<value value=\"7\" />\n\t\t\t\t\t\t\t<value value=\"8\" />\n\t\t\t\t\t\t\t<value value=\"9\" />\n\t\t\t\t\t\t</allowedValues>\n\t\t\t\t\t</parameter>\n\t\t\t\t\t<parameter uniqueID=\"UID_PARAM_240002\" access=\"readWrite\">\n\t\t\t\t\t\t<label lang=\"en\">RS232 rate</label>\n\t\t\t\t\t\t<USINT />\n\t\t\t\t\t\t<denotation>\n\t\t\t\t\t\t\t<label lang=\"en\" />\n\t\t\t\t\t\t</denotation>\n\t\t\t\t\t\t<defaultValue value=\"3\" />\n\t\t\t\t\t\t<allowedValues>\n\t\t\t\t\t\t\t<range>\n\t\t\t\t\t\t\t\t<minValue value=\"0\" />\n\t\t\t\t\t\t\t\t<maxValue value=\"3\" />\n\t\t\t\t\t\t\t</range>\n\t\t\t\t\t\t\t<value value=\"0\" />\n\t\t\t\t\t\t\t<value value=\"1\" />\n\t\t\t\t\t\t\t<value value=\"2\" />\n\t\t\t\t\t\t\t<value value=\"3\" />\n\t\t\t\t\t\t</allowedValues>\n\t\t\t\t\t</parameter>\n\t\t\t\t\t<parameter uniqueID=\"UID_PARAM_6007\" access=\"readWriteInput\">\n\t\t\t\t\t\t<label lang=\"en\">Abort connection option code</label>\n\t\t\t\t\t\t<INT />\n\t\t\t\t\t\t<denotation>\n\t\t\t\t\t\t\t<label lang=\"en\" />\n\t\t\t\t\t\t</denotation>\n\t\t\t\t\t\t<defaultValue value=\"1\" />\n\t\t\t\t\t\t<allowedValues>\n\t\t\t\t\t\t\t<range>\n\t\t\t\t\t\t\t\t<minValue value=\"-32768\" />\n\t\t\t\t\t\t\t\t<maxValue value=\"32767\" />\n\t\t\t\t\t\t\t</range>\n\t\t\t\t\t\t\t<value value=\"0\" />\n\t\t\t\t\t\t\t<value value=\"1\" />\n\t\t\t\t\t\t\t<value value=\"2\" />\n\t\t\t\t\t\t\t<value value=\"3\" />\n\t\t\t\t\t\t</allowedValues>\n\t\t\t\t\t</parameter>\n\t\t\t\t\t<parameter uniqueID=\"UID_PARAM_605A\" access=\"readWriteInput\">\n\t\t\t\t\t\t<label lang=\"en\">Quick-Stop option code</label>\n\t\t\t\t\t\t<INT />\n\t\t\t\t\t\t<denotation>\n\t\t\t\t\t\t\t<label lang=\"en\" />\n\t\t\t\t\t\t</denotation>\n\t\t\t\t\t\t<defaultValue value=\"2\" />\n\t\t\t\t\t\t<allowedValues>\n\t\t\t\t\t\t\t<range>\n\t\t\t\t\t\t\t\t<minValue value=\"0\" />\n\t\t\t\t\t\t\t\t<maxValue value=\"8\" />\n\t\t\t\t\t\t\t</range>\n\t\t\t\t\t\t\t<value value=\"0\" />\n\t\t\t\t\t\t\t<value value=\"1\" />\n\t\t\t\t\t\t\t<value value=\"2\" />\n\t\t\t\t\t\t\t<value value=\"3\" />\n\t\t\t\t\t\t\t<value value=\"4\" />\n\t\t\t\t\t\t\t<value value=\"5\" />\n\t\t\t\t\t\t\t<value value=\"6\" />\n\t\t\t\t\t\t\t<value value=\"7\" />\n\t\t\t\t\t\t\t<value value=\"8\" />\n\t\t\t\t\t\t</allowedValues>\n\t\t\t\t\t</parameter>\n\t\t\t\t\t<parameter uniqueID=\"UID_PARAM_605B\" access=\"readWriteInput\">\n\t\t\t\t\t\t<label lang=\"en\">Shutdown option code</label>\n\t\t\t\t\t\t<INT />\n\t\t\t\t\t\t<denotation>\n\t\t\t\t\t\t\t<label lang=\"en\" />\n\t\t\t\t\t\t</denotation>\n\t\t\t\t\t\t<defaultValue value=\"0\" />\n\t\t\t\t\t\t<allowedValues>\n\t\t\t\t\t\t\t<range>\n\t\t\t\t\t\t\t\t<minValue value=\"0\" />\n\t\t\t\t\t\t\t\t<maxValue value=\"1\" />\n\t\t\t\t\t\t\t</range>\n\t\t\t\t\t\t\t<value value=\"0\" />\n\t\t\t\t\t\t\t<value value=\"1\" />\n\t\t\t\t\t\t</allowedValues>\n\t\t\t\t\t</parameter>\n\t\t\t\t\t<parameter uniqueID=\"UID_PARAM_605C\" access=\"readWriteInput\">\n\t\t\t\t\t\t<label lang=\"en\">Disable operation option code</label>\n\t\t\t\t\t\t<INT />\n\t\t\t\t\t\t<denotation>\n\t\t\t\t\t\t\t<label lang=\"en\" />\n\t\t\t\t\t\t</denotation>\n\t\t\t\t\t\t<defaultValue value=\"1\" />\n\t\t\t\t\t\t<allowedValues>\n\t\t\t\t\t\t\t<range>\n\t\t\t\t\t\t\t\t<minValue value=\"0\" />\n\t\t\t\t\t\t\t\t<maxValue value=\"1\" />\n\t\t\t\t\t\t\t</range>\n\t\t\t\t\t\t\t<value value=\"0\" />\n\t\t\t\t\t\t\t<value value=\"1\" />\n\t\t\t\t\t\t</allowedValues>\n\t\t\t\t\t</parameter>\n\t\t\t\t\t<parameter uniqueID=\"UID_PARAM_605D\" access=\"readWriteInput\">\n\t\t\t\t\t\t<label lang=\"en\">Halt option code</label>\n\t\t\t\t\t\t<INT />\n\t\t\t\t\t\t<denotation>\n\t\t\t\t\t\t\t<label lang=\"en\" />\n\t\t\t\t\t\t</denotation>\n\t\t\t\t\t\t<defaultValue value=\"1\" />\n\t\t\t\t\t\t<allowedValues>\n\t\t\t\t\t\t\t<range>\n\t\t\t\t\t\t\t\t<minValue value=\"1\" />\n\t\t\t\t\t\t\t\t<maxValue value=\"4\" />\n\t\t\t\t\t\t\t</range>\n\t\t\t\t\t\t\t<value value=\"1\" />\n\t\t\t\t\t\t\t<value value=\"2\" />\n\t\t\t\t\t\t\t<value value=\"3\" />\n\t\t\t\t\t\t\t<value value=\"4\" />\n\t\t\t\t\t\t</allowedValues>\n\t\t\t\t\t</parameter>\n\t\t\t\t\t<parameter uniqueID=\"UID_PARAM_605E\" access=\"readWriteInput\">\n\t\t\t\t\t\t<label lang=\"en\">Fault reaction option code</label>\n\t\t\t\t\t\t<INT />\n\t\t\t\t\t\t<denotation>\n\t\t\t\t\t\t\t<label lang=\"en\" />\n\t\t\t\t\t\t</denotation>\n\t\t\t\t\t\t<defaultValue value=\"2\" />\n\t\t\t\t\t\t<allowedValues>\n\t\t\t\t\t\t\t<range>\n\t\t\t\t\t\t\t\t<minValue value=\"0\" />\n\t\t\t\t\t\t\t\t<maxValue value=\"4\" />\n\t\t\t\t\t\t\t</range>\n\t\t\t\t\t\t\t<value value=\"0\" />\n\t\t\t\t\t\t\t<value value=\"1\" />\n\t\t\t\t\t\t\t<value value=\"2\" />\n\t\t\t\t\t\t\t<value value=\"3\" />\n\t\t\t\t\t\t\t<value value=\"4\" />\n\t\t\t\t\t\t</allowedValues>\n\t\t\t\t\t</parameter>\n\t\t\t\t\t<parameter uniqueID=\"UID_PARAM_6060\" access=\"readWriteInput\">\n\t\t\t\t\t\t<label lang=\"en\">Modes of operation</label>\n\t\t\t\t\t\t<SINT />\n\t\t\t\t\t\t<denotation>\n\t\t\t\t\t\t\t<label lang=\"en\" />\n\t\t\t\t\t\t</denotation>\n\t\t\t\t\t\t<defaultValue value=\"0\" />\n\t\t\t\t\t\t<allowedValues>\n\t\t\t\t\t\t\t<range>\n\t\t\t\t\t\t\t\t<minValue value=\"-6\" />\n\t\t\t\t\t\t\t\t<maxValue value=\"10\" />\n\t\t\t\t\t\t\t</range>\n\t\t\t\t\t\t\t<value value=\"1\" />\n\t\t\t\t\t\t\t<value value=\"3\" />\n\t\t\t\t\t\t\t<value value=\"6\" />\n\t\t\t\t\t\t\t<value value=\"8\" />\n\t\t\t\t\t\t\t<value value=\"9\" />\n\t\t\t\t\t\t\t<value value=\"10\" />\n\t\t\t\t\t\t\t<value value=\"-1\" />\n\t\t\t\t\t\t\t<value value=\"-2\" />\n\t\t\t\t\t\t\t<value value=\"-3\" />\n\t\t\t\t\t\t\t<value value=\"-4\" />\n\t\t\t\t\t\t</allowedValues>\n\t\t\t\t\t</parameter>\n\t\t\t\t\t<parameter uniqueID=\"UID_PARAM_607E\" access=\"readWriteInput\">\n\t\t\t\t\t\t<label lang=\"en\">Polarity</label>\n\t\t\t\t\t\t<USINT />\n\t\t\t\t\t\t<denotation>\n\t\t\t\t\t\t\t<label lang=\"en\" />\n\t\t\t\t\t\t</denotation>\n\t\t\t\t\t\t<defaultValue value=\"0x0\" />\n\t\t\t\t\t\t<allowedValues>\n\t\t\t\t\t\t\t<range>\n\t\t\t\t\t\t\t\t<minValue value=\"0\" />\n\t\t\t\t\t\t\t\t<maxValue value=\"255\" />\n\t\t\t\t\t\t\t</range>\n\t\t\t\t\t\t\t<value value=\"0xC0\" />\n\t\t\t\t\t\t\t<value value=\"0x80\" />\n\t\t\t\t\t\t\t<value value=\"0x40\" />\n\t\t\t\t\t\t\t<value value=\"0x0\" />\n\t\t\t\t\t\t</allowedValues>\n\t\t\t\t\t</parameter>\n\t\t\t\t\t<parameter uniqueID=\"UID_PARAM_6086\" access=\"readWriteInput\">\n\t\t\t\t\t\t<label lang=\"en\">Motion profile type</label>\n\t\t\t\t\t\t<INT />\n\t\t\t\t\t\t<denotation>\n\t\t\t\t\t\t\t<label lang=\"en\" />\n\t\t\t\t\t\t</denotation>\n\t\t\t\t\t\t<defaultValue value=\"0\" />\n\t\t\t\t\t\t<allowedValues>\n\t\t\t\t\t\t\t<range>\n\t\t\t\t\t\t\t\t<minValue value=\"-32768\" />\n\t\t\t\t\t\t\t\t<maxValue value=\"32767\" />\n\t\t\t\t\t\t\t</range>\n\t\t\t\t\t\t\t<value value=\"0\" />\n\t\t\t\t\t\t\t<value value=\"1\" />\n\t\t\t\t\t\t</allowedValues>\n\t\t\t\t\t</parameter>\n\t\t\t\t\t<parameter uniqueID=\"UID_PARAM_60F2\" access=\"readWriteInput\">\n\t\t\t\t\t\t<label lang=\"en\">Position option code</label>\n\t\t\t\t\t\t<UINT />\n\t\t\t\t\t\t<denotation>\n\t\t\t\t\t\t\t<label lang=\"en\" />\n\t\t\t\t\t\t</denotation>\n\t\t\t\t\t\t<defaultValue value=\"0x0000\" />\n\t\t\t\t\t\t<allowedValues>\n\t\t\t\t\t\t\t<range>\n\t\t\t\t\t\t\t\t<minValue value=\"0\" />\n\t\t\t\t\t\t\t\t<maxValue value=\"0x00C0\" />\n\t\t\t\t\t\t\t</range>\n\t\t\t\t\t\t\t<value value=\"0x0000\" />\n\t\t\t\t\t\t\t<value value=\"0x00C0\" />\n\t\t\t\t\t\t</allowedValues>\n\t\t\t\t\t</parameter>\n\t\t\t\t</parameterList>\n\t\t\t</ApplicationProcess>\n\t\t</ProfileBody>\n\t</ISO15745Profile>\n\t<ISO15745Profile>\n\t\t<ProfileHeader>\n\t\t\t<ProfileIdentification>CAN comm net profile</ProfileIdentification>\n\t\t\t<ProfileRevision>1</ProfileRevision>\n\t\t\t<ProfileName></ProfileName>\n\t\t\t<ProfileSource></ProfileSource>\n\t\t\t<ProfileClassID>CommunicationNetwork</ProfileClassID>\n\t\t\t<ISO15745Reference>\n\t\t\t\t<ISO15745Part>1</ISO15745Part>\n\t\t\t\t<ISO15745Edition>1</ISO15745Edition>\n\t\t\t\t<ProfileTechnology>CANopen</ProfileTechnology>\n\t\t\t</ISO15745Reference>\n\t\t</ProfileHeader>\n\t\t<ProfileBody xsi:type=\"ProfileBody_CommunicationNetwork_CANopen\" fileName=\"605.0161.01-O.xdd\" fileCreator=\"Dr. Fritz Faulhaber GmbH &amp; Co KG\" fileCreationDate=\"2024-11-08\" fileCreationTime=\"07:04:39\" fileModificationDate=\"2024-11-08\" fileModificationTime=\"07:04:39\" fileModifiedBy=\"Dr. Fritz Faulhaber GmbH &amp; Co KG\" fileVersion=\"1\" supportedLanguages=\"en\">\n\t\t\t<ApplicationLayers>\n\t\t\t\t<identity>\n\t\t\t\t\t<vendorID>327</vendorID>\n\t\t\t\t\t<productID>016101</productID>\n\t\t\t\t</identity>\n\t\t\t\t<CANopenObjectList>\n\t\t\t\t\t<CANopenObject index=\"1000\" name=\"Device type\" objectType=\"7\" dataType=\"0007\" accessType=\"ro\" defaultValue=\"0x420192\" PDOmapping=\"no\" />\n\t\t\t\t\t<CANopenObject index=\"1001\" name=\"Error register\" objectType=\"7\" dataType=\"0005\" accessType=\"ro\" PDOmapping=\"TPDO\" />\n\t\t\t\t\t<CANopenObject index=\"1003\" name=\"Pre-defined error field\" objectType=\"8\" subNumber=\"9\">\n\t\t\t\t\t\t<CANopenSubObject subIndex=\"00\" name=\"Number of errors\" objectType=\"7\" dataType=\"0005\" lowLimit=\"0\" highLimit=\"255\" accessType=\"rw\" defaultValue=\"0\" PDOmapping=\"no\" objFlags=\"0001\" />\n\t\t\t\t\t\t<CANopenSubObject subIndex=\"01\" name=\"Standard error field 1\" objectType=\"7\" dataType=\"0007\" accessType=\"ro\" defaultValue=\"0x0\" PDOmapping=\"no\" objFlags=\"0003\" />\n\t\t\t\t\t\t<CANopenSubObject subIndex=\"02\" name=\"Standard error field 2\" objectType=\"7\" dataType=\"0007\" accessType=\"ro\" defaultValue=\"0x0\" PDOmapping=\"no\" objFlags=\"0003\" />\n\t\t\t\t\t\t<CANopenSubObject subIndex=\"03\" name=\"Standard error field 3\" objectType=\"7\" dataType=\"0007\" accessType=\"ro\" defaultValue=\"0x0\" PDOmapping=\"no\" objFlags=\"0003\" />\n\t\t\t\t\t\t<CANopenSubObject subIndex=\"04\" name=\"Standard error field 4\" objectType=\"7\" dataType=\"0007\" accessType=\"ro\" defaultValue=\"0x0\" PDOmapping=\"no\" objFlags=\"0003\" />\n\t\t\t\t\t\t<CANopenSubObject subIndex=\"05\" name=\"Standard error field 5\" objectType=\"7\" dataType=\"0007\" accessType=\"ro\" defaultValue=\"0x0\" PDOmapping=\"no\" objFlags=\"0003\" />\n\t\t\t\t\t\t<CANopenSubObject subIndex=\"06\" name=\"Standard error field 6\" objectType=\"7\" dataType=\"0007\" accessType=\"ro\" defaultValue=\"0x0\" PDOmapping=\"no\" objFlags=\"0003\" />\n\t\t\t\t\t\t<CANopenSubObject subIndex=\"07\" name=\"Standard error field 7\" objectType=\"7\" dataType=\"0007\" accessType=\"ro\" defaultValue=\"0x0\" PDOmapping=\"no\" objFlags=\"0003\" />\n\t\t\t\t\t\t<CANopenSubObject subIndex=\"08\" name=\"Standard error field 8\" objectType=\"7\" dataType=\"0007\" accessType=\"ro\" defaultValue=\"0x0\" PDOmapping=\"no\" objFlags=\"0003\" />\n\t\t\t\t\t</CANopenObject>\n\t\t\t\t\t<CANopenObject index=\"1005\" name=\"COB-ID SYNC\" objectType=\"7\" dataType=\"0007\" lowLimit=\"1\" highLimit=\"4294967295\" accessType=\"rw\" defaultValue=\"0x80\" PDOmapping=\"no\" />\n\t\t\t\t\t<CANopenObject index=\"1008\" name=\"Manufacturer device name\" objectType=\"7\" dataType=\"0009\" accessType=\"const\" PDOmapping=\"no\" />\n\t\t\t\t\t<CANopenObject index=\"1009\" name=\"Manufacturer hardware version\" objectType=\"7\" dataType=\"0009\" accessType=\"const\" PDOmapping=\"no\" />\n\t\t\t\t\t<CANopenObject index=\"100A\" name=\"Manufacturer software version\" objectType=\"7\" dataType=\"0009\" accessType=\"const\" PDOmapping=\"no\" />\n\t\t\t\t\t<CANopenObject index=\"100C\" name=\"Guard time\" objectType=\"7\" dataType=\"0006\" lowLimit=\"0\" highLimit=\"65535\" accessType=\"rw\" defaultValue=\"0\" PDOmapping=\"no\" />\n\t\t\t\t\t<CANopenObject index=\"100D\" name=\"Life time f
